vi "Read Current.vi"(8 "error in (no error)":errorcluster, 10 "Channel (1: Channel 1)":i32(ring)=1 items=["Channel 1"=1, "Channel 2"=2, "Channel 3"=3], 11 "VISA resource name":refnum<visa-resource-name>) -> (0 "error out":errorcluster, 1 "Actual Current Level (A)":dbl format="%.2g", 3 "VISA resource name out":refnum<visa-resource-name>)   [LabVIEW 2010, in "Agilent U2722.lvlib"]
doc: "Returns the actual voltage level and actual current level for a desired channel."
uses:
  Agilent U2722.lvlib
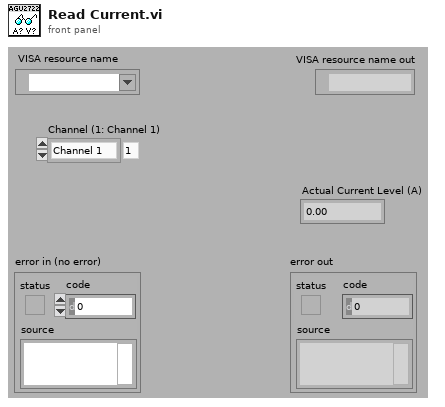
[diagram p1: front panel]
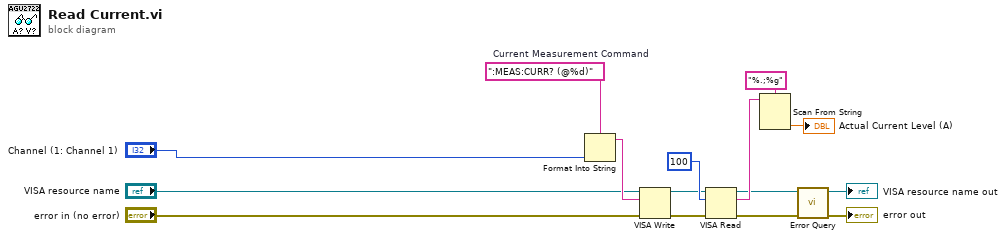
[diagram p0: block diagram]
diagram:
  w5 = ":MEAS:CURR? (@%d)"  # Current Measurement Command
  n1 = Format Into String(format string=w5, "Channel (1: Channel 1)") -> (resulting string=w4:string)  [unwired: 2 in, 1 out]
  n2 = VISA Write(VISA resource name="VISA resource name", write buffer=w4, error in (no error)="error in (no error)") -> (VISA resource name out=w10:refnum<visa-resource-name>, error out=w9:errorcluster)  [unwired: 1 out]
  n3 = VISA Read(VISA resource name=w10, byte count=u32 100, error in (no error)=w9) -> (VISA resource name out=w7:refnum<visa-resource-name>, read buffer=w12:string, error out=w6:errorcluster)  [unwired: 1 out]
  n4 = Scan From String(format string="%.;%g", input string=w12) -> (output 1=→"Actual Current Level (A)":dbl)  [unwired: 3 in, 3 out]
  n5 = call "Error Query.vi"("error in (no error)"=w6, "VISA resource name"=w7) -> ("error out"=→"error out":errorcluster, "VISA resource name out"=→"VISA resource name out":refnum<visa-resource-name>)  [unwired: 6 in, 2 out]
